vi "IMAGE_TRANSFER_MODE_PARAM.vi"() -> (0 "IMAGE_TRANSFER_MODE_PARAM":T1 {"wMode" items=["IMAGE_TRANSFER_MODE_STANDARD"=0, "IMAGE_TRANSFER_MODE_SCALED_XY_8BIT"=1, "IMAGE_TRANSFER_MODE_CUTOUT_XY_8BIT"=2, "IMAGE_TRANSFER_MODE_FULL_RGB_24BIT"=3, "IMAGE_TRANSFER_MODE_BIN_SCALED_8BIT_BW"=4, "IMAGE_TRANSFER_MODE_BIN_SCALED_8BIT_COLOR"=5, "IMAGE_TRANSFER_MODE_TEST_ONLY"=32768]}, 1 "IMAGE_TRANSFER_MODE_PARAM_RAW":T2 {"wMode" items=["IMAGE_TRANSFER_MODE_STANDARD"=0, "IMAGE_TRANSFER_MODE_SCALED_XY_8BIT"=1, "IMAGE_TRANSFER_MODE_CUTOUT_XY_8BIT"=2, "IMAGE_TRANSFER_MODE_FULL_RGB_24BIT"=3, "IMAGE_TRANSFER_MODE_BIN_SCALED_8BIT_BW"=4, "IMAGE_TRANSFER_MODE_BIN_SCALED_8BIT_COLOR"=5, "IMAGE_TRANSFER_MODE_TEST_ONLY"=32768]}, 2 "Length":u16, 3 "Raw_Length":u16)   [LabVIEW 2020, in "SDK.lvlib" / "Structures.lvlib"]
doc: "Use this template to build a VI to use as a subVI."
uses:
  Structures.lvlib
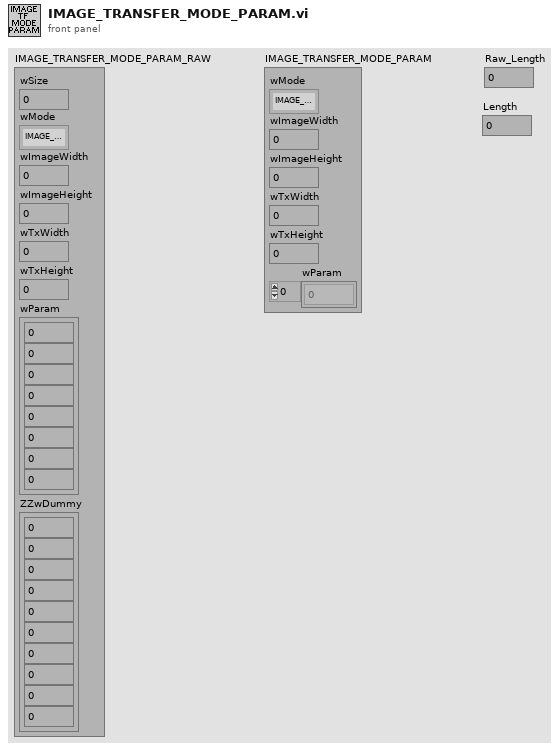
[diagram p1: front panel]
types:
  T1 = cluster{"wMode":u16, "wImageWidth":u16, "wImageHeight":u16, "wTxWidth":u16, "wTxHeight":u16, "wParam":u16[]}
  T2 = cluster{"wSize":u16, "wMode":u16, "wImageWidth":u16, "wImageHeight":u16, "wTxWidth":u16, "wTxHeight":u16, "wParam":cluster{u16, u16, u16, u16, u16, u16, u16, u16}, "ZZwDummy":cluster{u16, u16, u16, u16, u16, u16, u16, u16, u16, u16}}
  T3 = cluster{u16, u16, u16, u16, u16, u16, u16, u16, u16, u16}
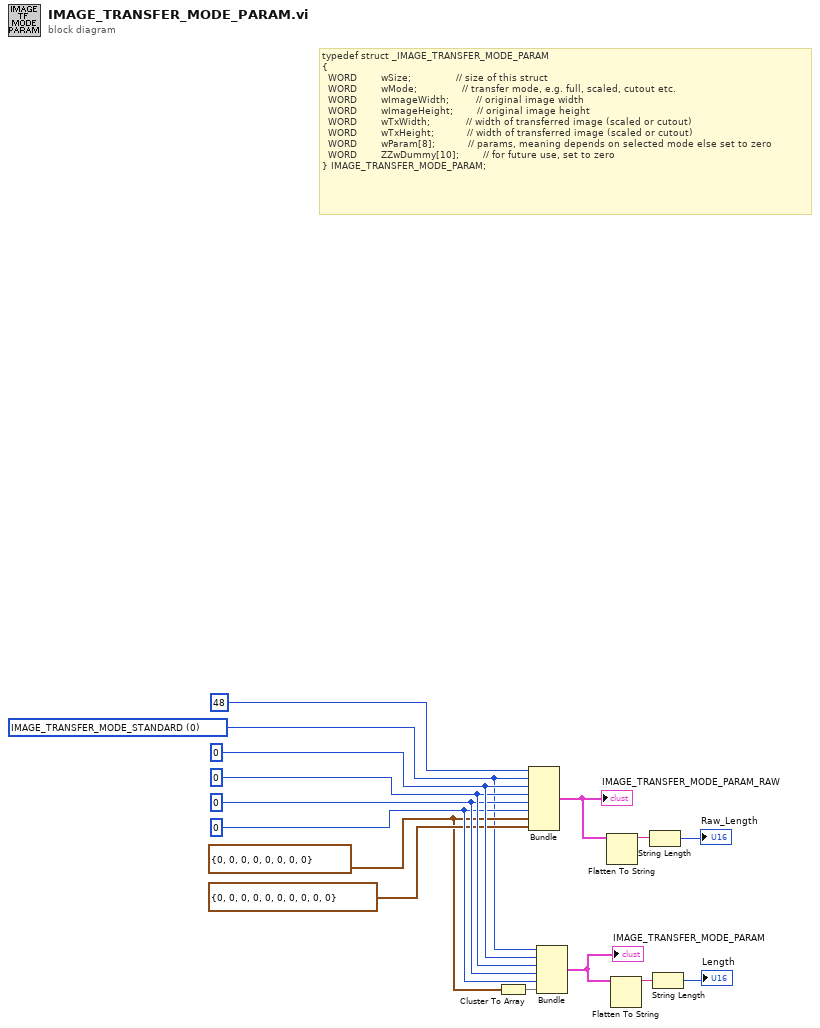
[diagram p0: block diagram]
diagram:
  w1 = u16 0 items=["IMAGE_TRANSFER_MODE_STANDARD"=0, "IMAGE_TRANSFER_MODE_SCALED_XY_8BIT"=1, "IMAGE_TRANSFER_MODE_CUTOUT_XY_8BIT"=2, "IMAGE_TRANSFER_MODE_FULL_RGB_24BIT"=3, "IMAGE_TRANSFER_MODE_BIN_SCALED_8BIT_BW"=4, "IMAGE_TRANSFER_MODE_BIN_SCALED_8BIT_COLOR"=5, "IMAGE_TRANSFER_MODE_TEST_ONLY"=32768] ("wMode")
  w2 = cluster{u16, u16, u16, u16, u16, u16, u16, u16} {0, 0, 0, 0, 0, 0, 0, 0} ("wParam")
  w6 = u16 0 ("wTxHeight")
  w7 = u16 0 ("wTxWidth")
  w8 = u16 0 ("wImageHeight")
  w9 = u16 0 ("wImageWidth")
  # "typedef struct _IMAGE_TRANSFER_MODE_PARAM\n{\n  WORD        wSize;               // size of this struct\n  WORD        wMode;               // transfer mode, e.g. full, scaled, cutout etc.\n  WORD        wImageWidth;         // original image width\n  WORD        wImageHeight;        // original image height\n  WORD        wTxWidth;            // width of transferred image (scaled or cutout)\n  WORD        wTxHeight;           // width of transferred image (scaled or cutout)\n  WORD        wParam[8];           // params, meaning depends on selected mode else set to zero\n  WORD        ZZwDummy[10];        // for future use, set to zero\n} IMAGE_TRANSFER_MODE_PARAM;"
  n1 = Cluster To Array(cluster=w2) -> (array=w3:u16[])
  n2 = Bundle("wSize"=u16 48, "wMode"=w1, "wImageWidth"=w9, "wImageHeight"=w8, "wTxWidth"=w7, "wTxHeight"=w6, "wParam"=w2, "ZZwDummy"=T3 {0, 0, 0, 0, 0, 0, 0, 0, 0, 0}) -> (w10:T2)  [unwired: 1 in]
  "IMAGE_TRANSFER_MODE_PARAM_RAW" <- w10
  n3 = Bundle("wMode"=w1, "wImageWidth"=w9, "wImageHeight"=w8, "wTxWidth"=w7, "wTxHeight"=w6, "wParam"=w3) -> (w5:T1)  [unwired: 1 in]
  "IMAGE_TRANSFER_MODE_PARAM" <- w5
  n4 = Flatten To String(anything=w10) -> (data string=w14:string)  [unwired: 3 in, 2 out]
  n5 = Flatten To String(anything=w5) -> (data string=w15:string)  [unwired: 3 in, 2 out]
  n6 = String Length(string=w14) -> (length=→"Raw_Length":i32)
  n7 = String Length(string=w15) -> (length=→"Length":i32)
